vi "dfd_FLP IIR II.vi"(7 "x":dbl format="%.2f", 9 "states in":dbl[](array[numeric]) format="%.2f", 10 "coefficients a":dbl[](array[numeric]) format="%.2f", 11 "coefficients b":dbl[](array[numeric]) format="%.2f") -> (1 "states out":dbl[](array[numeric]) format="%.2f", 2 "w":dbl, 3 "y":dbl format="%.2f")   [LabVIEW 2017, in "NI_DigFilter_FXP.lvlib"]
uses:
  <vilib>/addons/Digital Filter Design/NI_DigFilter_FXP.lvlib
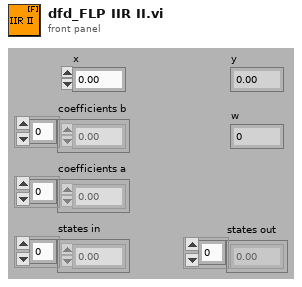
[diagram p1: front panel]
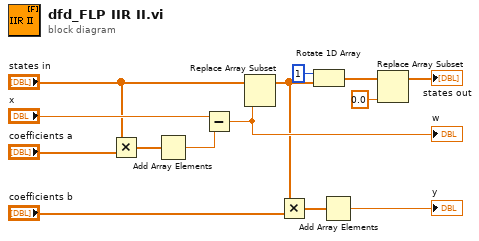
[diagram p0: block diagram]
diagram:
  n1 = Multiply(x="states in", y="coefficients a") -> (x*y=w9:dbl[])
  n2 = Add Array Elements(numeric array=w9) -> (sum=w8:dbl)
  n3 = Subtract(x="x", y=w8) -> (x-y=w7:dbl)
  "w" <- w7
  n4 = Replace Array Subset(array="states in", new element=w7) -> (w6:dbl[])  [unwired: 1 in]
  n5 = Multiply(x=w6, y="coefficients b") -> (x*y=w11:dbl[])
  n6 = Rotate 1D Array(1:w6, 2:1 ("n")) -> (0:w5:dbl[])
  n7 = Add Array Elements(numeric array=w11) -> (sum=→"y":dbl)
  n8 = Replace Array Subset(array=w5, new element=0.0 ("new element/subarray")) -> (→"states out":dbl[])  [unwired: 1 in]
